vi "UpdateElement(Single).vi"(7 "Qualified Name":string, 8 "error in (no error)":errorcluster, 9 "Value":string, 10 "Key":string, 11 "SMOConfigManager in":refnum<class "ConfigManager.lvclass">) -> (0 "error out":errorcluster, 3 "SMOConfigManager out":refnum<class "ConfigManager.lvclass">)   [LabVIEW 2013, in "SMOConfig.lvlib" / "ConfigManager.lvclass"]
uses:
  ConfigManager.lvclass
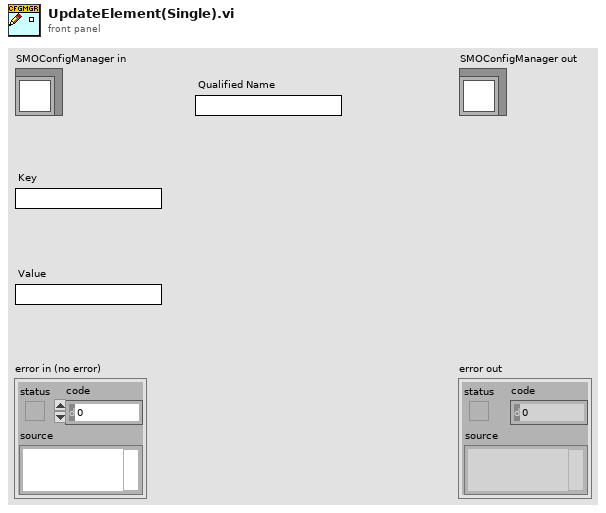
[diagram p1: front panel]
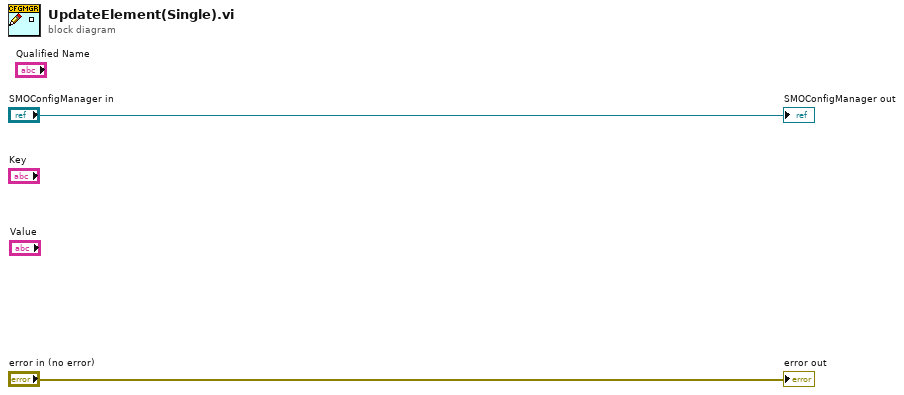
[diagram p0: block diagram]
diagram:
  "error out" <- "error in (no error)"
  "SMOConfigManager out" <- "SMOConfigManager in"
